vi "Receive Control Key Up Event.vi"(8 "error in (no error)":errorcluster, 10 "ControlKeyUpMsg":refnum<class "ControlKeyUpMsg.lvclass">, 11 "TopButton In":refnum<class "TopButton.lvclass">) -> (0 "error out":errorcluster, 3 "TopButton Out":refnum<class "TopButton.lvclass">)   [LabVIEW 2017, in "TopButton.lvlib" / "TopButton.lvclass"]
doc: "<License>\nCopyright © 2017 Composed Systems, LLC | All rights reserved\nwww.composed.io\n\nAuthor: Ethan Stern <ethan.stern@composed.io>\n\nThis software is provided \"AS IS\" WITHOUT WARRANTIES, either express or implied, AND IS FOR EDUCATIONAL PURPOSES ONLY.\n</License>"
uses:
  <vilib>/gpm_packages/TestSystem/Views/TopButton/TopButton/TopButton.lvclass
  <vilib>/gpm_packages/@cs/mva-viewable/Source/ActorEvents/IEventAggregator Messages/ControlKeyUpMsg/ControlKeyUpMsg.lvclass
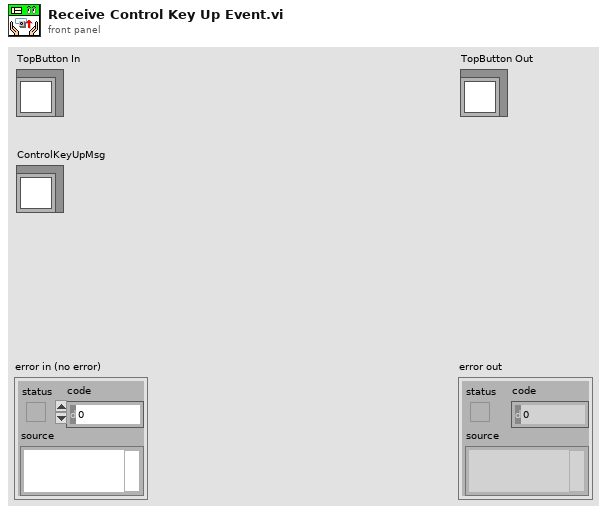
[diagram p1: front panel]
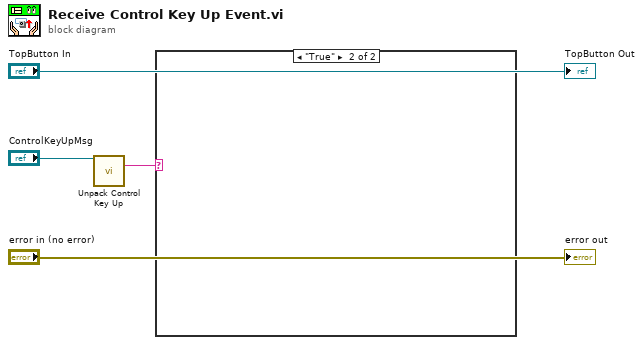
[diagram p0: block diagram]
diagram:
  n1 = call <vilib>:"Unpack Control Key Up.vi"("ControlKeyUpMsg"="ControlKeyUpMsg") -> ("Control Label"=w3:string)  [unwired: 8 in, 6 out]
  n2 = case shown="\"True\"" w3 {
    frame "False", Default {
    }
    frame "True" {
    }
  }
  "error out" <- "error in (no error)"
  "TopButton Out" <- "TopButton In"
